vi "Application Version.vi"() -> ()   [LabVIEW 2021]
panel:
  out "version":string
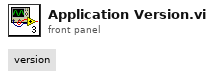
[diagram p1: front panel]
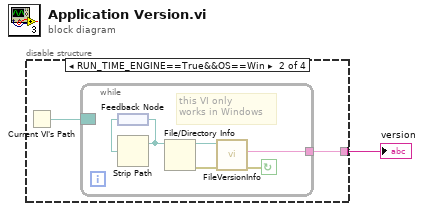
[diagram p0: block diagram]
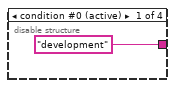
[diagram p2: hidden frame]
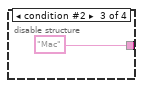
[diagram p3: hidden frame]
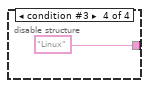
[diagram p4: hidden frame]
diagram:
  n1 = disable-structure "Conditional Disable Structure" shown="RUN_TIME_ENGINE==True&&OS==Win" {
    disable-tunnel: ["development" w3 "Mac" "Linux"] -> w1
    frame condition #0 (active) {
    }
    frame condition #1 {
      n2 = Current VI's Path() -> (path=w4:path)
      n3 = while {
        border: w4 -> [_]
        tunnel: [w5] -> w3
        stop <- w9 continue-if-true
        # "this VI only \nworks in Windows"
        n4 = feedback #1() -> (w8:path)
        n5 = Strip Path(path=w8) -> (stripped path=w7:path)  [unwired: 1 out]
        n6 = feedback-in #1(w7) -> ()
        n7 = File/Directory Info(path=w7) -> (path out=w6:path, error out=w10:errorcluster)  [unwired: 1 in, 5 out]
        n8 = call <vilib>:"FileVersionInfo.vi"("error in (no error)"=w10, "Application Path in"=w6) -> ("error out"=w9:errorcluster, "File Version Info"=w5:string)  [unwired: 6 in, 2 out]
      }
    }
    frame condition #2 {
    }
    frame condition #3 {
    }
  }
  "version" <- w1
